vi "是否合法.vi"(8 "列":dbl, 9 "行":dbl, 11 "地图":dbl[][](array[numeric])) -> (2 "元素":dbl, 3 "是否合法":bool)   [LabVIEW 2023]
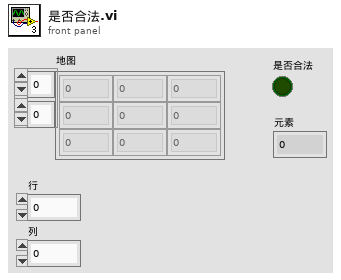
[diagram p1: front panel]
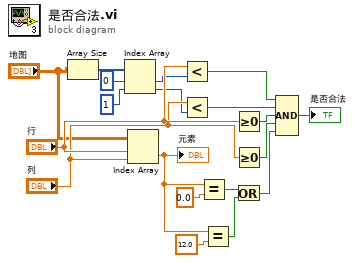
[diagram p0: block diagram]
diagram:
  n1 = Array Size(array="地图") -> (size(s)=w6:i32[])
  n2 = Index Array(array=w6, index #1=0 ("索引"), index #2=1 ("索引")) -> (element #1=w2:i32, element #2=w1:i32)
  n3 = Index Array(array="地图", index (row)="行", index (col)="列") -> (element=w19:dbl)
  "元素" <- w19
  n4 = Less?(x="行", y=w2) -> (x < y?=w14:bool)
  n5 = Less?(x="列", y=w1) -> (x < y?=w13:bool)
  n6 = Equal?(x=w19, y=0.0) -> (x = y?=w15:bool)
  n7 = Equal?(x=w19, y=12.0) -> (x = y?=w16:bool)
  n8 = Greater Or Equal To 0?(x="行") -> (x >= 0?=w12:bool)
  n9 = Greater Or Equal To 0?(x="列") -> (x >= 0?=w11:bool)
  n10 = Or(x=w15, y=w16) -> (x .or. y?=w10:bool)
  n11 = Compound Arithmetic op=AND ("复合运算")(w14, w13, w12, w11, w10) -> (→"是否合法":bool)
